vi "RangeMeasureLimitClose.vi"(8 "error in":errorcluster, 11 "RangeMeasureLimit":refnum<class "RangeMeasureLimit.lvclass">) -> (0 "error out":errorcluster)   [LabVIEW 2021, in "ProligentXMLGenerator.lvlib" / "RangeMeasureLimit.lvclass"]
uses:
  RangeMeasureLimit.lvclass
  RangeMeasureLimit.lvclass/RangeMeasureLimit.ctl
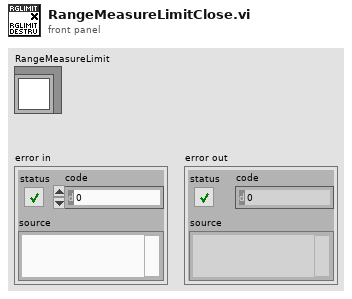
[diagram p1: front panel]
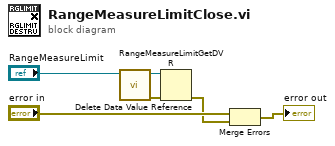
[diagram p0: block diagram]
diagram:
  n1 = call "RangeMeasureLimitGetDVR.vi"("RangeMeasureLimit"="RangeMeasureLimit") -> ("error out"=w3:errorcluster, "DVRReference"=w4:refnum<data-value>)  [unwired: 9 in]
  n2 = Delete Data Value Reference(data value reference=w4, error in=w3) -> (error out=w2:errorcluster)  [unwired: 1 out]
  n3 = Merge Errors("error in", w2) -> (→"error out":errorcluster)
